vi "Clear Report.vi"(0 "report in":refnum<class "NI_Standard Report.lvclass">, 11 "error in (no error)":errorcluster) -> (4 "report out":refnum<class "NI_Standard Report.lvclass">, 15 "error out":errorcluster)   [LabVIEW 2017, in "NI_Standard Report.lvclass"]
doc: "Clears the report of all text, headers, footers, and formatting information."
uses:
  <vilib>/Utility/NIReport.llb/Standard Report/NI_Standard Report.lvclass
  <vilib>/Utility/NIReport.llb/Standard Report/NI_Standard Report.lvclass/NI_Standard Report.ctl
  <vilib>/Utility/NIReport.llb/NI_ReportGenerationCore.lvlib
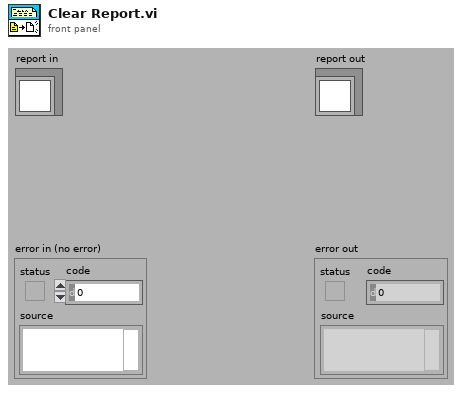
[diagram p1: front panel]
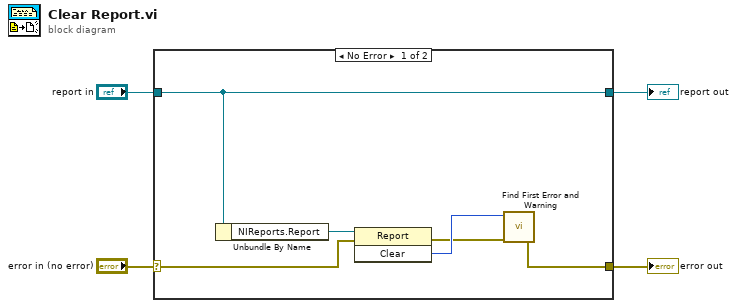
[diagram p0: block diagram]
diagram:
  n1 = case shown="No Error" "error in (no error)" {
    selector: "error in (no error)" -> [w7 w12]
    tunnel: [w6 w12] -> w3
    tunnel: [w5 w11] -> w1
    tunnel: "report in" -> [w5 w11]
    frame No Error {
      n2 = Unbundle By Name(w5) -> ("NIReports.Report"=w8:refnum<k7>)
      n3 = invoke class="Report" method="Clear"(reference=w8, error in=w7) -> (error out=w9:errorcluster, "Clear"=w10:i32)  [unwired: 1 in, 1 out]
      n4 = call <vilib>:"Find First Error and Warning.vi"("error in (no error)"=w9, "error code"=w10) -> ("error out"=w6:errorcluster)  [unwired: 1 in, 4 out]
    }
    frame Error {
    }
  }
  "error out" <- w3
  "report out" <- w1
